vi "example_00_architecture.vi"() -> ()   [LabVIEW 2015]
uses:
  functional/public/_controls/event_functional.ctl
  functional/public/_controls/event_functional_command.ctl
  functional/public/interface/interface.lvclass
  functional/functional.lvlib
panel:
  out "stopped":bool
  in  "launch":bool
  in  "stop":bool
  out "error out":errorcluster
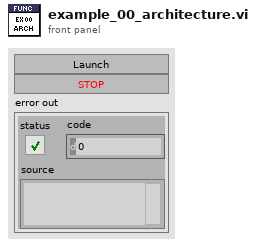
[diagram p1: front panel]
types:
  T1 = typedef "functional.lvlib/event_functional.ctl" = cluster{"command":T2, "data":variant}
  T2 = typedef "functional.lvlib/event_functional_command.ctl" = enum16{"<command_functional>", "--high-level", "stop", "update_hmi_references", "load_interface", "--functional", "<null>"}
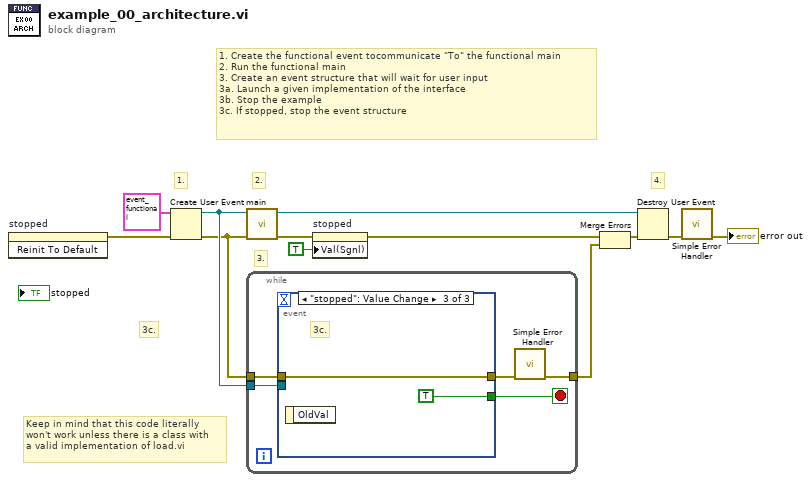
[diagram p0: block diagram]
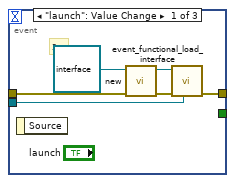
[diagram p2: hidden frame]
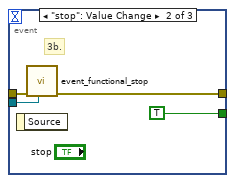
[diagram p3: hidden frame]
diagram:
  # "1. Create the functional event tocommunicate \"To\" the functional main\n2. Run the functional main\n3. Create an event structure that will wait for user input\n3a. Launch a given implementation of the interface\n3b. Stop the example\n3c. If stopped, stop the event structure"
  # "Keep in mind that this code literally\nwon't work unless there is a class with\na valid implementation of load.vi"
  # "4."
  # "3c."
  # "3."
  # "2."
  # "1."
  n1 = invoke on="stopped" class="Bool (strict)" method="Reinit To Default"() -> (error out=w4:errorcluster)  [unwired: 3 in, 2 out]
  n2 = Create User Event(user event datatype=T1 {"command"=enum."<command_functional>", "data"=variant} ("functional"), error in=w4) -> (user event=w6:refnum<user-event>, error out=w5:errorcluster)
  n3 = call "main.vi"("error in (no error)"=w5, "common"=w6) -> ("error out"=w2:errorcluster)  [unwired: 9 in]
  n4 = while {
    tunnel: w5 -> [w15]
    tunnel: [w12] -> w8
    tunnel: w6 -> [w13]
    stop <- w16 stop-if-true
    n5 = event shown="[2] \"stopped\": Value Change" {
      selector: _ -> [_ _ _]
      dyn-events: _ -> [_ _ _]
      timeout: _ -> [_ _ _]
      tunnel: [_ TRUE TRUE] -> w16
      tunnel: w15 -> [w21 w25 w27]
      tunnel: [w22 w24 w27] -> w14
      tunnel: w13 -> [w19 w23 _]
      event "launch": Value Change {
        # "3a."
        n6 = event-data() -> ()  [unwired: 1 in, 1 out]
        n7 = call-dynamic "new.vi"("error in (no error)"=w21, "interface in"=refnum<class "interface.lvclass"> refnum) -> ("error out"=w20:errorcluster, "interface out"=w17:refnum<class "interface.lvclass">)  [unwired: 8 in]
        n8 = call "event_functional_load_interface.vi"("functional"=w19, "error in (no error)"=w20, "interface"=w17) -> ("error out"=w22:errorcluster)  [unwired: 8 in]
      }
      event "stop": Value Change {
        # "3b."
        n9 = event-data() -> ()  [unwired: 1 in, 1 out]
        n10 = call "event_functional_stop.vi"("functional"=w23, "error in (no error)"=w25) -> ("error out"=w24:errorcluster)  [unwired: 9 in]
      }
      event "stopped": Value Change {
        # "3c."
        n11 = event-data() -> ()  [unwired: 1 in, 1 out]
      }
    }
    n12 = call <vilib>:"Simple Error Handler.vi"("error in (no error)"=w14) -> ("error out"=w12:errorcluster)  [unwired: 4 in, 4 out]
  }
  n13 = property on="stopped" class="Bool (strict)"(error in=w2, "Val(Sgnl)"=TRUE ("Value (Signaling)")) -> (error out=w1:errorcluster)  [unwired: 1 in, 1 out]
  n14 = Merge Errors(w1, w8) -> (w10:errorcluster)
  n15 = Destroy User Event(user event=w6, error in=w10) -> (error out=w9:errorcluster)
  n16 = call <vilib>:"Simple Error Handler.vi"("error in (no error)"=w9) -> ("error out"=→"error out":errorcluster)  [unwired: 4 in, 4 out]
